vi "Main.vi"() -> ()   [LabVIEW 2014]
uses:
  <vilib>/imath/engines/lvmath2/RunTimeEngine/BuiltInFunctions/sort/NIMS_[1o]_sort(RRowV,I32,Str).vi
  <instcachedir>/0/NIMS_[1o]_sort(RRowV,I32,Str)_5666ACD9F309401B9D8935C6ABFD847C.lvgen/NIMS_[1o]_sort(RRowV,I32,Str)_5666ACD9F309401B9D8935C6ABFD847C_000.vi
  <vilib>/imathl/engines/lvmath/Functions/Error Handling/Create Error.vi
  <vilib>/imath/engines/lvmath2/RunTimeEngine/BuiltInFunctions/length/NIMS_length(GV).vi
  <instcachedir>/0/NIMS_length(GV)_08A3D13377FD4E4B96F5795FBF3698FA.lvgen/NIMS_length(GV)_08A3D13377FD4E4B96F5795FBF3698FA_000.vi
  <vilib>/imath/engines/lvmath2/RunTimeEngine/RangeToken/NIMS_Range.vi
  <instcachedir>/0/NIMS_Range_9BCE657718DF4976A877346C61F22738.lvgen/NIMS_Range_9BCE657718DF4976A877346C61F22738_000.vi
  <vilib>/imath/engines/lvmath2/RunTimeSupport/NIMS_Error if Not Equal.vi
  <instcachedir>/0/NIMS_Error if Not Equal_8A0E9F659B9142D69417CC259581C4FD.lvgen/NIMS_Error if Not Equal_8A0E9F659B9142D69417CC259581C4FD_001.vi
  <vilib>/imath/engines/lvmath2/RunTimeEngine/IndexRead/NIMS V(V).vi
  <instcachedir>/0/NIMS V(V)_298D9CB7BFEB42B8BC8D9C3C28AE8C70.lvgen/NIMS V(V)_298D9CB7BFEB42B8BC8D9C3C28AE8C70_000.vi
  <vilib>/imath/engines/lvmath2/RunTimeEngine/BuiltInFunctions/mean/NIMS_RS=mean(RV,I32).vi
  <vilib>/imath/engines/lvmath2/RunTimeEngine/ErrorHandling/NIMS_Create Error From Enums.vi
  <vilib>/imath/engines/lvmath2/RunTimeEngine/BuiltInFunctions/std/NIMS_std(GV,RV).vi
  <instcachedir>/0/NIMS_std(GV,RV)_28FF1B2340C147788D324E9DB4F24E07.lvgen/NIMS_std(GV,RV)_28FF1B2340C147788D324E9DB4F24E07_001.vi
  <vilib>/imath/engines/lvmath2/RunTimeEngine/BuiltInFunctions/findnz/NIMS_[1o]_findnz(GRowV).vi
  <instcachedir>/0/NIMS_[1o]_findnz(GRowV)_09DEEFCD766A4095B33095726AFD3FF8.lvgen/NIMS_[1o]_findnz(GRowV)_09DEEFCD766A4095B33095726AFD3FF8_000.vi
  <vilib>/imath/engines/lvmath2/RunTimeEngine/BuiltInFunctions/is_empty/NIMS_is_empty(GV).vi
  <instcachedir>/0/NIMS_is_empty(GV)_FC7E7C3D9544432CB6AA2416ADCF6D56.lvgen/NIMS_is_empty(GV)_FC7E7C3D9544432CB6AA2416ADCF6D56_000.vi
  <instcachedir>/0/NIMS_length(GV)_08A3D13377FD4E4B96F5795FBF3698FA.lvgen/NIMS_length(GV)_08A3D13377FD4E4B96F5795FBF3698FA_002.vi
  <vilib>/imath/engines/lvmath2/RunTimeEngine/RangeToken/NIMS_Range_R2 - Integer.vi
  <instcachedir>/0/NIMS_Range_R2 - Integer_2D1304BAF97744E0A293025746CBADFC.lvgen/NIMS_Range_R2 - Integer_2D1304BAF97744E0A293025746CBADFC_000.vi
  <vilib>/imath/engines/lvmath2/RunTimeEngine/CommandStatement/MC_CommandStatement_break.vi
  <vilib>/imath/engines/lvmath2/RunTimeEngine/IndexRead/NIMS V(S).vi
  <instcachedir>/0/NIMS V(S)_0488751826AF41519A22953C041130DC.lvgen/NIMS V(S)_0488751826AF41519A22953C041130DC_002.vi
  <vilib>/imath/engines/lvmath2/RunTimeEngine/BuiltInFunctions/min/1 input/NIMS_min(RV).vi
  <instcachedir>/0/NIMS_min(RV)_EE2DD3E2888846108C5160A664B67832.lvgen/NIMS_min(RV)_EE2DD3E2888846108C5160A664B67832_002.vi
  <vilib>/imath/engines/lvmath2/RunTimeEngine/IndexRead/NIMS V(R2).vi
  <instcachedir>/0/NIMS V(R2)_C76619605A0E4E9F8B2FA9389712AC47.lvgen/NIMS V(R2)_C76619605A0E4E9F8B2FA9389712AC47_000.vi
  <instcachedir>/0/NIMS_min(RV)_EE2DD3E2888846108C5160A664B67832.lvgen/NIMS_min(RV)_EE2DD3E2888846108C5160A664B67832_000.vi
  <vilib>/imath/engines/lvmath2/RunTimeEngine/BuiltInFunctions/max/1 input/NIMS_max(RV).vi
  <instcachedir>/0/NIMS_max(RV)_237633DB1D604D5BA7001287DF3C7957.lvgen/NIMS_max(RV)_237633DB1D604D5BA7001287DF3C7957_000.vi
  <vilib>/imath/engines/lvmath2/RunTimeEngine/RowToken/NIMS_RowToken_M_SorRV.vi
  <instcachedir>/0/NIMS_RowToken_M_SorRV_FBF65B742C8C47AA9A456487F0E79BF9.lvgen/NIMS_RowToken_M_SorRV_FBF65B742C8C47AA9A456487F0E79BF9_001.vi
  <vilib>/imath/engines/lvmath2/RunTimeEngine/NodeEndStatement/NIMS_NodeEndStatement_Get Vector.vi
  <instcachedir>/0/NIMS_NodeEndStatement_Get Vector_00D1625602D843AD9D7EC134A9EC13A2.lvgen/NIMS_NodeEndStatement_Get Vector_00D1625602D843AD9D7EC134A9EC13A2_002.vi
  <vilib>/imath/engines/lvmath/Functions/Error Handling/MergeErrorsWrapper.vi
  <vilib>/imath/engines/lvmath2/RunTimeEngine/NodeEndStatement/NIMS_NodeEndStatement_Output.vi
  <instcachedir>/0/NIMS_NodeEndStatement_Output_53EC0D466D134D7ABD903AC30B43404B.lvgen/NIMS_NodeEndStatement_Output_53EC0D466D134D7ABD903AC30B43404B_004.vi
  <instcachedir>/0/NIMS_NodeEndStatement_Output_53EC0D466D134D7ABD903AC30B43404B.lvgen/NIMS_NodeEndStatement_Output_53EC0D466D134D7ABD903AC30B43404B_001.vi
  <vilib>/imath/engines/lvmath2/RunTimeEngine/ErrorHandling/NIMS_Finalize Error.vi
  <vilib>/Analysis/NI_AALBase.lvlib
  <vilib>/gmath/NI_Gmath.lvlib
panel:
  out "Waveform Graph":dbl[][](graph)
  out "locs":i32[][](array[numeric])
  out "Resampled Data":dbl[][](graph)
  out "RMS":dbl[][](graph)
  in  "Input File":path=path "C:/Users/Dany/Documents/GitHub/PQ/data.tdms"
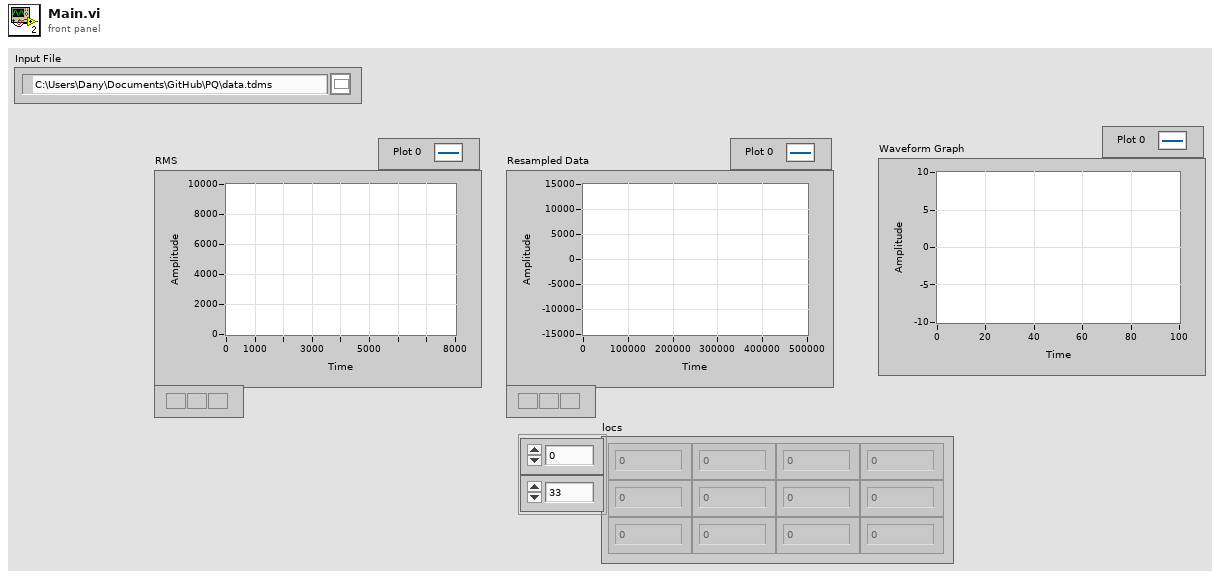
[diagram p1: front panel]
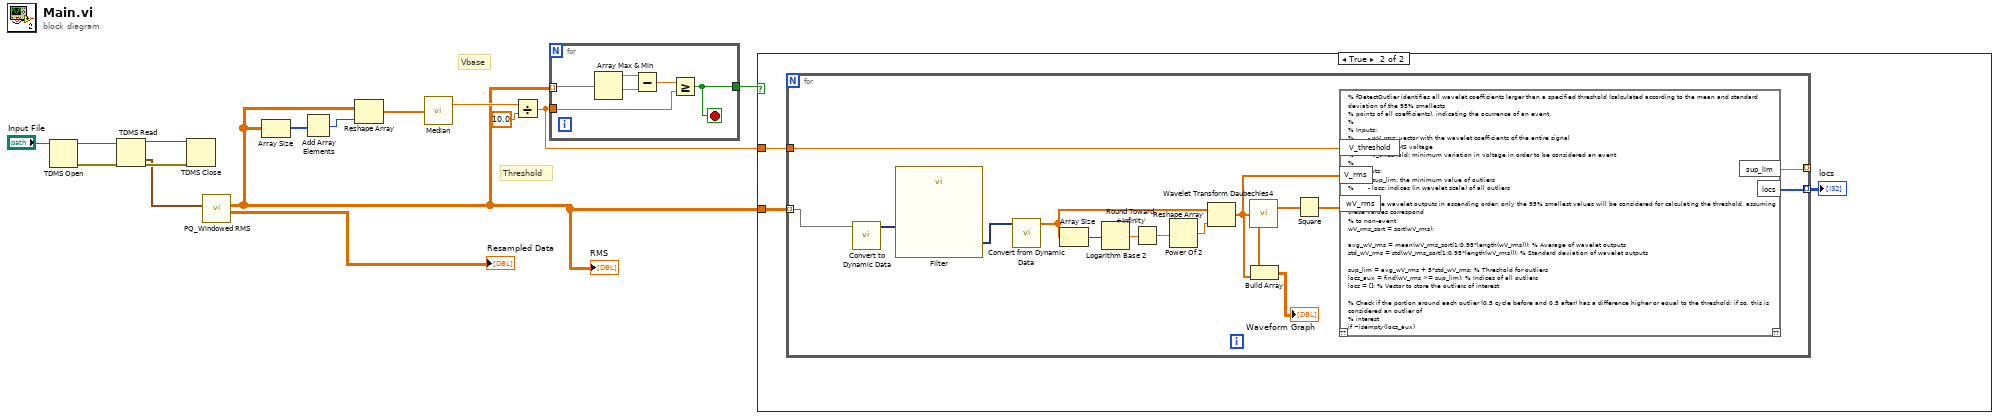
[diagram p0: block diagram]
diagram:
  # "Threshold"
  # "Vbase"
  n1 = TDMS Open(11:"Input File") -> (0:w14:errorcluster, 3:w15:refnum<k34>)  [unwired: 6 in]
  n2 = TDMS Read(0:w15, 11:w14) -> (4:w13:refnum<k34>, 10:w10:waveform(dbl)[], 15:w12:errorcluster)  [unwired: 6 in, 3 out]
  n3 = TDMS Close(8:w12, 11:w13) -> ()  [unwired: 2 out]
  n4 = call "PQ_Windowed RMS.vi"("data"=w10) -> ("Resampled Data"=→"Resampled Data":dbl[][], "RMS"=w3:dbl[][])  [unwired: 9 in]
  "RMS" <- w3
  n5 = Array Size(array=w3) -> (size(s)=w1:i32[])
  n6 = Add Array Elements(numeric array=w1) -> (sum=w2:i32)
  n7 = Reshape Array(w3, w2) -> (w4:dbl[])
  n8 = call <vilib>:"Median.vi"("X"=w4) -> ("median"=w6:dbl)  [unwired: 1 out]
  n9 = Divide(x=w6, y=10.0) -> (x/y=w5:dbl)
  n10 = for {
    tunnel: w3 -> [w21] mode=indexing
    tunnel: [w17] -> w8
    tunnel: w5 -> [w16]
    stop <- w17 stop-if-true
    n11 = Array Max & Min(array=w21) -> (max value=w20:dbl, min value=w19:dbl)  [unwired: 2 out]
    n12 = Subtract(x=w20, y=w19) -> (x-y=w18:dbl)
    n13 = Greater Or Equal?(x=w18, y=w16) -> (x >= y?=w17:bool)
  }
  n14 = case shown="True" w8 {
    tunnel: w3 -> [_ w24]
    tunnel: w5 -> [_ w23]
    frame False {
    }
    frame True {
      n15 = for {
        tunnel: w24 -> [w31] mode=indexing
        tunnel: [w38] -> _ mode=indexing
        tunnel: [w37] -> w22 mode=indexing
        tunnel: w23 -> [w36]
        n16 = call "Convert to Dynamic Data"("Array"=w31) -> ("Dynamic Data Type"=w30:dynamicdata)  [unwired: 3 in]
        n17 = call "Filter"("Signal"=w30) -> ("Filtered Signal"=w29:dynamicdata)  [unwired: 9 in, 1 out]
        n18 = call "Convert from Dynamic Data"("Dynamic Data Type"=w29) -> ("Array"=w28:dbl[])  [unwired: 3 in]
        n19 = Array Size(array=w28) -> (size(s)=w35:i32)
        n20 = Logarithm Base 2(1:w35) -> (0:w34:dbl)
        n21 = Round Toward +Infinity(x=w34) -> (ceil(x): smallest int >= x=w33:dbl)
        n22 = Power Of 2(x=w33) -> (2^x=w32:dbl)
        n23 = Reshape Array(w28, w32) -> (w26:dbl[])
        n24 = call <vilib>:"Wavelet Transform Daubechies4.vi"("X"=w26) -> ("Wavelet Daubechies4 {X}"=w27:dbl[])  [unwired: 1 out]
        n25 = Build Array(w27, w26) -> (→"Waveform Graph":dbl[][])
        n26 = Square(x=w27) -> (x^2=w39:dbl[])
        n27 = mathscript code="% fDetectOutlier identifies all wavelet coefficients larger than a specified threshold (calculated according to the mean and standard deviation of the 95% smallests\n% points of all coefficients), indicating the ocurrence of an event.\n%\n% Inputs:\n%       - wV_rms: vector with the wavelet coefficients of the entire signal\n%       - V_rms: RMS voltage\n%       - V_threshold: minimum variation in voltage in order to be considered an event\n%\n% Outputs:\n%       - sup_lim: the minimum value of outliers\n%       - locs: indices (in wavelet scale) of all outliers\n\n% Order the wavelet outputs in ascending order; only the 95% smallest values will be considered for calculating the threshold, assuming these values correspond\n% to non-event\nwV_rms_sort = sort(wV_rms); \n\navg_wV_rms = mean(wV_rms_sort(1:0.95*length(wV_rms))); % Average of wavelet outputs\nstd_wV_rms = std(wV_rms_sort(1:0.95*length(wV_rms))); % Standard deviation of wavelet outputs\n\nsup_lim = avg_wV_rms + 5*std_wV_rms; % Threshold for outliers\nlocs_aux = find(wV_rms >= sup_lim); % Indices of all outliers\nlocs = []; % Vector to store the outliers of interest\n\n% Check if the portion around each outlier (0.5 cycle before and 0.5 after) has a difference higher or equal to the threshold; if so, this is considered an outlier of\n% interest\nif ~isempty(locs_aux)\n\n    for k = 1:length(locs_aux)\n        range_low = min([2*locs_aux(k),64]); range_high = min([length(V_rms)-2*locs_aux(k),64]);\n        debug = max(V_rms(2*locs_aux(k)-range_low+1:2*locs_aux(k)+range_high)) - min(V_rms(2*locs_aux(k)-range_low+1:2*locs_aux(k)+range_high));\n        if max(V_rms(2*locs_aux(k)-range_low+1:2*locs_aux(k)+range_high)) - min(V_rms(2*locs_aux(k)-range_low+1:2*locs_aux(k)+range_high)) >= V_threshold\n            locs = [locs, locs_aux(k)];\n        end\n    end\nend"("wV_rms"=w39, "V_threshold"=w36, "V_rms"=w26) -> ("sup_lim"=w38:dbl, "locs"=w37:i32[])  [unwired: 1 in, 1 out]
      }
      "locs" <- w22
    }
  }
